vi "Read Subscriber List.vi"(11 "Topic in":refnum<class "Topic.lvclass">) -> (2 "Subscriber Policy List":T1[](array[typedef]))   [LabVIEW 2015, in "Mediator.lvlib" / "Topic.lvclass"]
doc: "<License>\nCopyright © 2017 Composed Systems, LLC | All rights reserved\nwww.composed.io\n\nAuthor: Ethan Stern <ethan.stern@composed.io>\n\nThis software is provided \"AS IS\" WITHOUT WARRANTIES, either express or implied, AND IS FOR EDUCATIONAL PURPOSES ONLY.\n</License>"
uses:
  Topic.lvclass
  IMediator/ISubscriptionPolicy/ISubscriptionPolicy Reference.ctl
  IMediator/ISubscriptionPolicy/ISubscriptionPolicy.lvclass
  Topic.lvclass/Topic.ctl
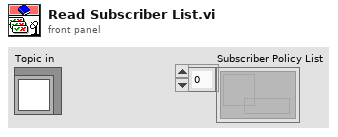
[diagram p1: front panel]
types:
  T1 = typedef "IMediator.lvlib/ISubscriptionPolicy.lvclass/ISubscriptionPolicy Reference.ctl" = refnum<data-value>
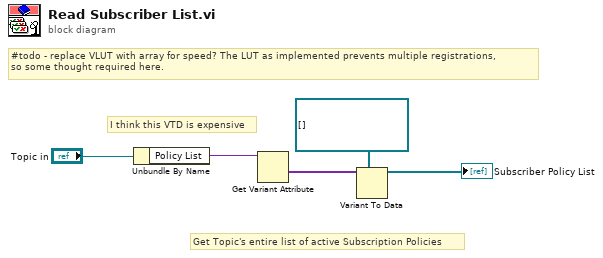
[diagram p0: block diagram]
diagram:
  # "I think this VTD is expensive"
  # "#todo - replace VLUT with array for speed? The LUT as implemented prevents multiple registrations,\nso some thought required here."
  # "Get Topic's entire list of active Subscription Policies"
  n1 = Unbundle By Name("Topic in") -> ("Policy List"=w5:variant)
  n2 = Get Variant Attribute(Variant=w5) -> (values=w1:variant[])  [unwired: 3 in, 3 out]
  n3 = Variant To Data(type=T1[] [] ("Topic Enqueuer"), Variant=w1) -> (data=→"Subscriber Policy List":T1[])  [unwired: 1 in, 1 out]
